vi "Lockin_Amplifier_diag_fast.vi"(0 "Refresh in (s)":dbl, 1 "dt":dbl, 5 "mean":dbl, 7 "Continous Lock-in":bool, 9 "Ref_MLD measurement":dbl[][](array[numeric]), 11 "Second":bool, 12 "Number of samples":i16, 14 "Sampling frequency":dbl) -> (4 "Result 2":dbl, 6 "Result":dbl)   [LabVIEW 2015]
uses:
  <vilib>/express/express arith-compare/Formula/XNode/ExpressFormulaBlockNode.xnode
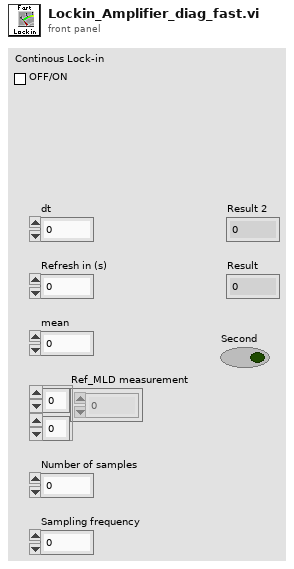
[diagram p1: front panel]
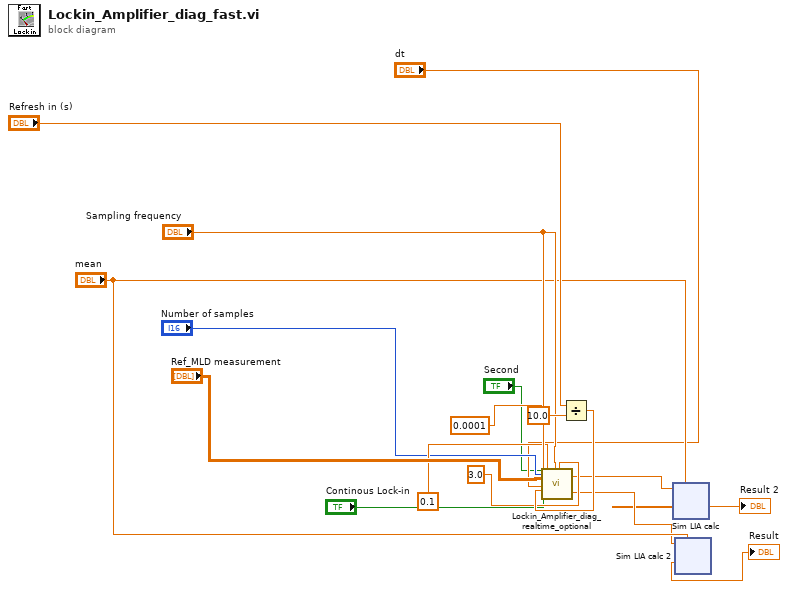
[diagram p0: block diagram]
diagram:
  n1 = Divide(x="Refresh in (s)", y=10.0) -> (x/y=w17:dbl)
  n2 = call "Lockin_Amplifier_diag_realtime_optional.vi"("Second"="Second", "Sample Number"="Number of samples", "all rows"="Ref_MLD measurement", "Cutoff Frequency"="Sampling frequency", "dt"="dt", "Window (s)"=w17, "Continous Lock-in"="Continous Lock-in", "Resolution"=0.0001, "averaging time"=0.1, "Sampling Freq"="Sampling frequency", "tolerance (Deviation)"=3.0 ("Window (s)")) -> ("dLD_RMS"=w9:dbl, "LD_RMS"=w7:dbl)  [unwired: 10 in, 5 out]
  n3 = xnode "Sim LIA calc"("X1"=w7, "X2"="mean") -> ("Result"=→"Result 2":dbl)  [unwired: 1 in, 1 out]
  n4 = xnode "Sim LIA calc 2"("X1"=w9, "X2"="mean") -> ("Result"=→"Result":dbl)  [unwired: 1 in, 1 out]
